vi "download_calibration_pv.vi"(8 "configuration":u64, 9 "port":u16, 10 "host":string, 11 "path in":path=path "hl2ss_ulm.dll") -> (1 "error":bool, 2 "calibration":T1, 3 "path out":path)   [LabVIEW 2023]
panel:
  in  "calibration":T1
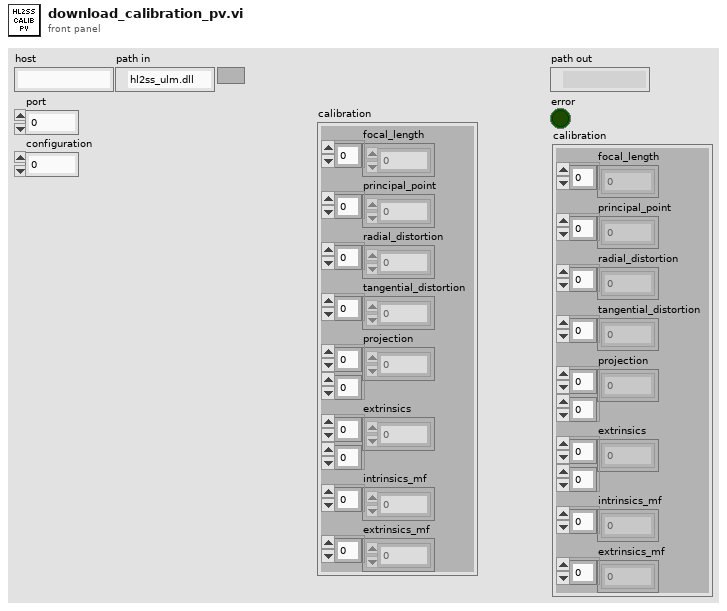
[diagram p1: front panel]
types:
  T1 = cluster{"focal_length":sgl[], "principal_point":sgl[], "radial_distortion":sgl[], "tangential_distortion":sgl[], "projection":sgl[][], "extrinsics":sgl[][], "intrinsics_mf":sgl[], "extrinsics_mf":sgl[]}
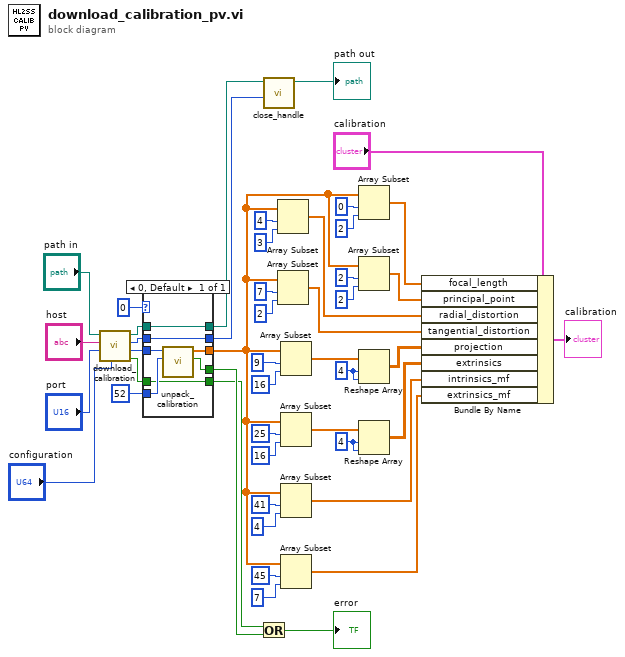
[diagram p0: block diagram]
diagram:
  w4 = 4 ("dimension size")
  w5 = 4 ("dimension size")
  n1 = call "download_calibration.vi"("configuration"="configuration", "port"="port", "host"="host", "path in"="path in") -> ("error"=w33:bool, "calibration"=w42:u64, "calibration_handle"=w40:u64, "path out"=w41:path)  [unwired: 4 in]
  n2 = case shown="0, Default" u64 0 ("configuration") {
    tunnel: 52 ("element_count") -> [w54]
    tunnel: w42 -> [w53]
    tunnel: w41 -> [w52]
    tunnel: w40 -> [w51]
    tunnel: [w52] -> w39
    tunnel: [w51] -> w38
    tunnel: [w50] -> w29
    tunnel: [w49] -> w37
    tunnel: [w48] -> w34
    tunnel: w33 -> [w48]
    frame 0, Default {
      n3 = call "unpack_calibration.vi"("element_count"=w54, "calibration"=w53) -> ("error"=w49:bool, "calibration"=w50:sgl[])  [unwired: 8 in]
    }
  }
  n4 = Or(x=w34, y=w37) -> (x .or. y?=→"error":bool)
  n5 = call "close_handle.vi"("handle"=w38, "path in"=w39) -> ("path out"=→"path out":path)  [unwired: 9 in]
  n6 = Array Subset(array=w29, index=4, length=3) -> (w10:sgl[])
  n7 = Array Subset(array=w29, index=7, length=2) -> (w9:sgl[])
  n8 = Array Subset(array=w29, index=9, length=16) -> (w6:sgl[])
  n9 = Array Subset(array=w29, index=25, length=16) -> (w3:sgl[])
  n10 = Array Subset(array=w29, index=41, length=4) -> (w7:sgl[])
  n11 = Array Subset(array=w29, index=45, length=7) -> (w8:sgl[])
  n12 = Array Subset(array=w29, index=0, length=2) -> (w12:sgl[])
  n13 = Array Subset(array=w29, index=2, length=2) -> (w11:sgl[])
  n14 = Reshape Array(w6, w5, w5) -> (w2:sgl[][])
  n15 = Reshape Array(w3, w4, w4) -> (w1:sgl[][])
  n16 = Bundle By Name(cluster="calibration", "focal_length"=w12, "principal_point"=w11, "radial_distortion"=w10, "tangential_distortion"=w9, "projection"=w2, "extrinsics"=w1, "intrinsics_mf"=w7, "extrinsics_mf"=w8) -> (→"calibration":T1)
